vi "set constant value.vi"(8 "error in":errorcluster, 9 "data to set":variant, 10 "control name":string, 11 "vi in":refnum<vi>) -> (0 "error out":errorcluster, 3 "vi out":refnum<vi>)   [LabVIEW 2013, in "NISE Tools Scripting.lvlib"]
uses:
  NISE Tools Scripting.lvlib
  <vilib>/Utility/traverseref.llb/TRef TravTarget.ctl
  <vilib>/Utility/traverseref.llb/VI Scripting - Traverse.lvlib
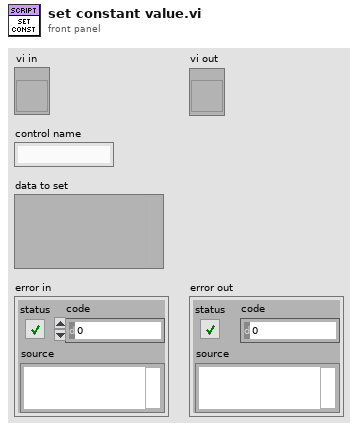
[diagram p1: front panel]
types:
  T1 = typedef "TRef TravTarget.ctl" = enum16{"FP", "BD", "Other"}
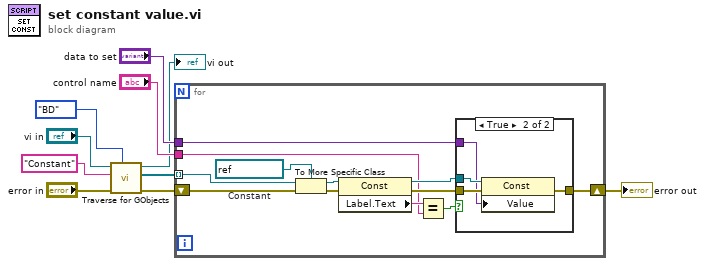
[diagram p0: block diagram]
diagram:
  n1 = call <vilib>:"Traverse for GObjects.vi"("Traverse Target"=TRef_TravTarget."BD", "error in (no error)"="error in", "Class Name"="Constant", "VI Refnum"="vi in") -> ("error out"=w6:errorcluster, "References"=w7:refnum<vi>[], "dup VI Refnum"=→"vi out":refnum<vi>)  [unwired: 4 in, 1 out]
  n2 = for {
    shift-right: [w15] -> w8
    shift-left: w6 -> [w22]
    tunnel: w7 -> [w21] mode=indexing
    tunnel: "control name" -> [w12]
    tunnel: "data to set" -> [w11]
    w20 = refnum<vi> refnum  # Constant
    n3 = To More Specific Class(target class=w20, reference=w21, error in=w22) -> (specific class reference=w19:refnum<vi>, error out=w18:errorcluster)
    n4 = property class="Const"(reference=w19, error in=w18) -> (reference out=w13:refnum<vi>, error out=w14:errorcluster, "Label.Text"=w17:string)
    n5 = Equal?(x=w17, y=w12) -> (x = y?=w16:bool)
    n6 = case shown="True" w16 {
      tunnel: [w23 w25] -> w15
      tunnel: w14 -> [w23 w27]
      tunnel: w13 -> [_ w26]
      tunnel: w11 -> [_ w24]
      frame False {
      }
      frame True {
        n7 = property class="Const"(reference=w26, error in=w27, "Value"=w24) -> (error out=w25:errorcluster)  [unwired: 1 out]
      }
    }
  }
  "error out" <- w8
